vi "Open.vi"(7 "Allow multiple opens?":bool, 8 "error in (no error)":errorcluster, 10 "Channel Names":tag[](array[tag])) -> (0 "error out":errorcluster, 3 "AO (N Samples) Ref Out":T1)   [LabVIEW 2021, in "AO Block.lvlib"]
doc: "Opens a reference to analog output block write channel (ConnectorA/AO0). You must open a reference before you write values to the analog output block write channel."
uses:
  <vilib>/myRIO/Instrument Drivers/Onboard IO/AO Block/AO Block.lvlib
  <vilib>/myRIO/Instrument Drivers/Onboard IO/AO Block/typedefs/AO Block Reference.ctl
  <vilib>/myRIO/Common/Instrument Driver Framework/Utilities/typedefs/myRIO Generic Hardware Reference.ctl
  <vilib>/myRIO/Common/Instrument Driver Framework/Utilities/typedefs/Hardware Version Enum.ctl
  <vilib>/myRIO/Common/Instrument Driver Framework/Utilities/typedefs/myRIO v1.0 Reference.ctl
  <vilib>/myRIO/Common/Instrument Driver Framework/Utilities/typedefs/Generic FPGA Reference.ctl
  <vilib>/myRIO/Common/Instrument Driver Framework/myRIO v1.0/AO Block/typedefs/AO Block Channels List.ctl
  <vilib>/myRIO/Common/Instrument Driver Framework/myRIO v1.0/AO Block/typedefs/AO Block Channels Enum.ctl
  <vilib>/myRIO/Common/Instrument Driver Framework/Utilities/typedefs/Analog Scaling Constants.ctl
  <vilib>/userdefined/High Color/nirio_resource_hc.ctl
panel:
  # "AO (N Samples) Open"
  # "Opens a reference to the myRIO hardware and configures the AO Block Reference with channels to be written"
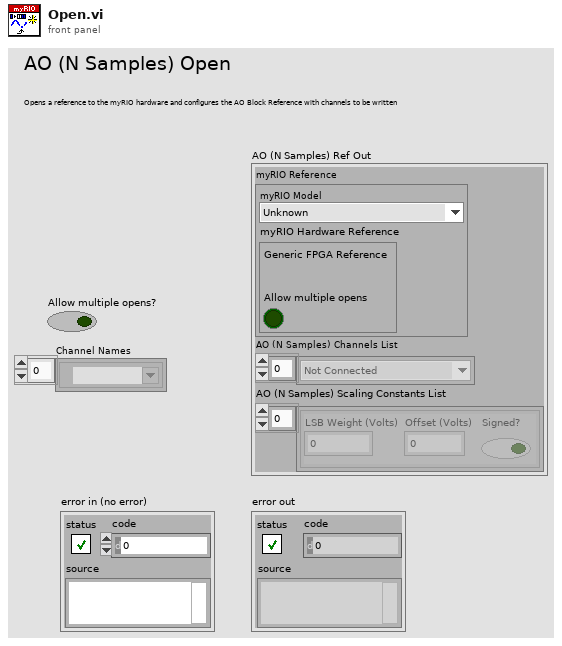
[diagram p1: front panel]
types:
  T1 = typedef "AO Block.lvlib/AO Block Reference.ctl" = cluster{"myRIO Reference":T2, "AO (N Samples) Channels List":T6, "AO (N Samples) Scaling Constants List":T8[]}
  T2 = typedef "myRIO Generic Hardware Reference.ctl" = cluster{"myRIO Model":T3, "myRIO Hardware Reference":T4}
  T3 = typedef "Hardware Version Enum.ctl" = enum16{"Unknown", "myRIO-1900", "myRIO-1950", "roboRIO", "NI ELVIS RIO CM", "ELVIS III"}
  T4 = typedef "myRIO v1.0 Reference.ctl" = cluster{"Generic FPGA Reference":T5, "Allow multiple opens":bool}
  T5 = typedef "Generic FPGA Reference.ctl" = refnum<k20>
  T6 = typedef "AO Block Channels List.ctl" = T7[]
  T7 = typedef "AO Block Channels Enum.ctl" = enum16{"Not Connected", "A/AO0 (N Samples)", "A/AO1 (N Samples)", "B/AO0 (N Samples)", "B/AO1 (N Samples)"}
  T8 = typedef "Analog Scaling Constants.ctl" = cluster{"LSB Weight (Volts)":dbl, "Offset (Volts)":dbl, "Signed?":bool}
  T9 = typedef "nirio_resource_hc.ctl" = tag
  T10 = typedef "Analog Scaling Constants List.ctl" = T8[]
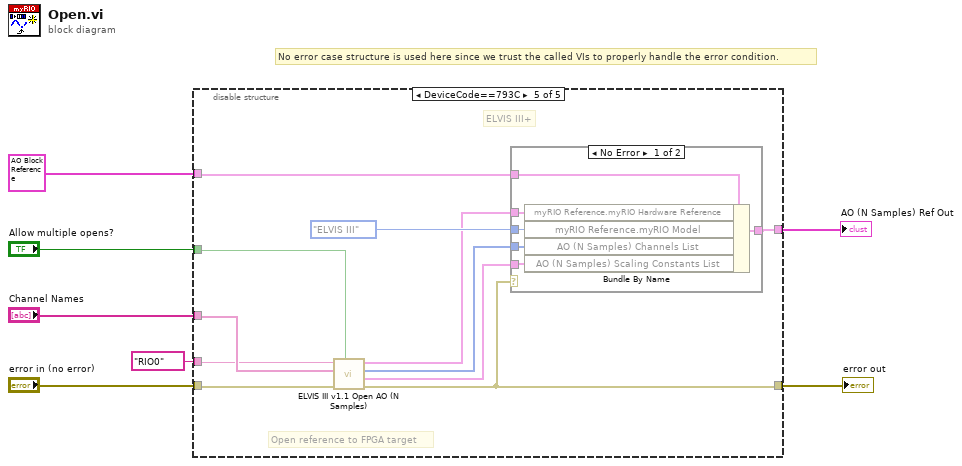
[diagram p0: block diagram]
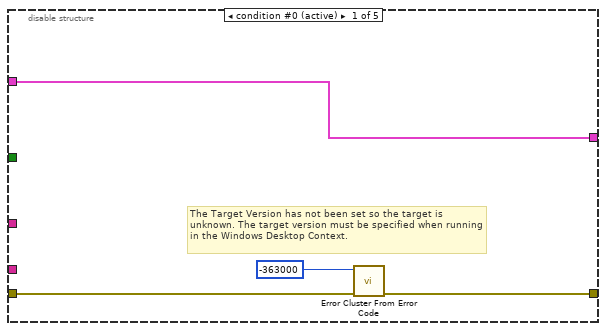
[diagram p2: hidden frame]
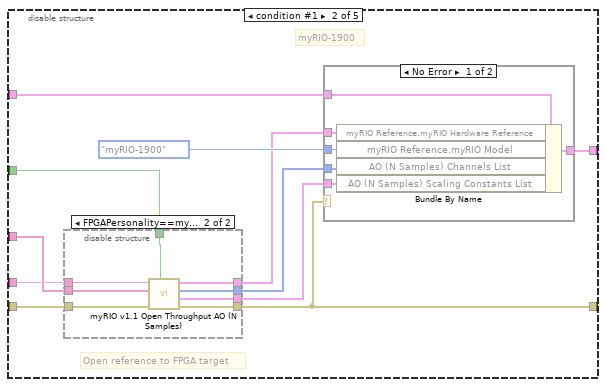
[diagram p3: hidden frame]
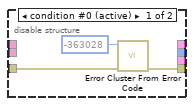
[diagram p4: hidden frame]
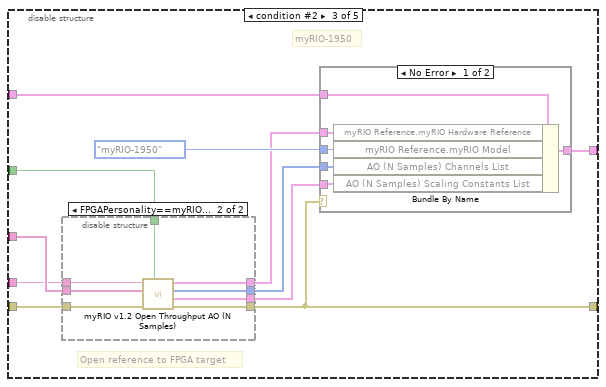
[diagram p6: hidden frame]
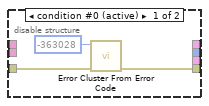
[diagram p7: hidden frame]
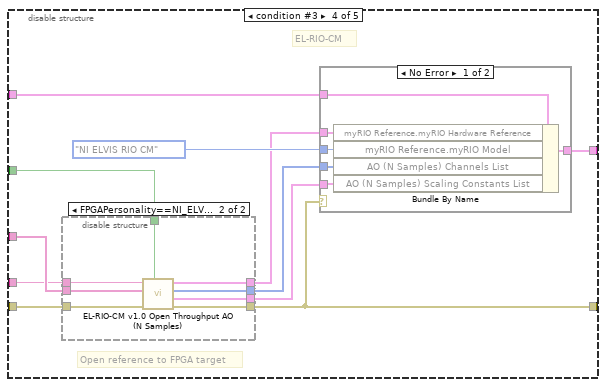
[diagram p9: hidden frame]
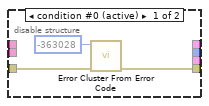
[diagram p10: hidden frame]
diagram:
  # "No error case structure is used here since we trust the called VIs to properly handle the error condition."
  n1 = disable-structure shown="DeviceCode==793C" {
    disable-tunnel: [w11 w14 w44 w73 w100] -> w5
    disable-tunnel: "Channel Names" -> [_ w22 w51 w80 w103]
    disable-tunnel: "Allow multiple opens?" -> [_ w18 w50 w79 w104]
    disable-tunnel: [w8 w21 w49 w78 w99] -> w4
    disable-tunnel: "error in (no error)" -> [w10 w19 w47 w76 w101]
    disable-tunnel: T1 {"myRIO Reference"={"myRIO Model"=enum."Unknown", "myRIO Hardware Reference"={"Generic FPGA Reference"=refnum, "Allow multiple opens"=FALSE}}, "AO (N Samples) Channels List"=[], "AO (N Samples) Scaling Constants List"=[]} ("AO (N Samples) Write Ref Out") -> [w8 w17 w46 w75 w105]
    disable-tunnel: T9 "RIO0" ("Resource name") -> [_ w15 w45 w74 w102]
    frame condition #0 (active) {
      # "The Target Version has not been set so the target is unknown. The target version must be specified when running in the Windows Desktop Context."
      n2 = call <vilib>:"Error Cluster From Error Code.vi"("error in (no error)"=w10, "error code (0)"=-363000) -> ("error out"=w11:errorcluster)  [unwired: 7 in]
    }
    frame condition #1 {
      # "myRIO-1900"
      # "Open reference to FPGA target"
      n3 = disable-structure shown="FPGAPersonality==myRIO_FP_Throughput" {
        disable-tunnel: w22 -> [_ w31]
        disable-tunnel: w19 -> [w24 w30]
        disable-tunnel: w18 -> [_ w33]
        disable-tunnel: [_ w28] -> w16
        disable-tunnel: w15 -> [_ w32]
        disable-tunnel: [w23 w26] -> w14
        disable-tunnel: [_ w29] -> w13
        disable-tunnel: [_ w27] -> w12
        frame condition #0 (active) {
          n4 = call <vilib>:"Error Cluster From Error Code.vi"("error in (no error)"=w24, "error code (0)"=-363028) -> ("error out"=w23:errorcluster)  [unwired: 7 in]
        }
        frame condition #1 {
          n5 = call <vilib>:"myRIO v1.1 Open Throughput AO (N Samples).vi"("Allow multiple opens?"=w33, "error in (no error)"=w30, "Channel Names"=w31, "Resource name"=w32) -> ("error out"=w26:errorcluster, "AO (N Samples) Scale Constants List"=w27:T10, "AO (N Samples) Channel List"=w28:T6, "myRIO Ref Out"=w29:T4)  [unwired: 4 in]
        }
      }
      n6 = case shown="No Error" w14 {
        tunnel: [w39 w40] -> w21
        tunnel: Hardware_Version_Enum."myRIO-1900" ("Hardware Version Enum") -> [w38 _]
        tunnel: w17 -> [w37 w40]
        tunnel: w16 -> [w36 _]
        tunnel: w13 -> [w35 _]
        tunnel: w12 -> [w34 _]
        frame No Error {
          n7 = Bundle By Name(cluster=w37, "myRIO Reference.myRIO Hardware Reference"=w35, "myRIO Reference.myRIO Model"=w38, "AO (N Samples) Channels List"=w36, "AO (N Samples) Scaling Constants List"=w34) -> (w39:T1)
        }
        frame Error {
        }
      }
    }
    frame condition #2 {
      # "myRIO-1950"
      # "Open reference to FPGA target"
      n8 = disable-structure shown="FPGAPersonality==myRIO_FP_Throughput" {
        disable-tunnel: w51 -> [_ w60]
        disable-tunnel: w50 -> [_ w62]
        disable-tunnel: w47 -> [w53 w59]
        disable-tunnel: w45 -> [_ w61]
        disable-tunnel: [w52 w55] -> w44
        disable-tunnel: [_ w58] -> w43
        disable-tunnel: [_ w57] -> w42
        disable-tunnel: [_ w56] -> w41
        frame condition #0 (active) {
          n9 = call <vilib>:"Error Cluster From Error Code.vi"("error in (no error)"=w53, "error code (0)"=-363028) -> ("error out"=w52:errorcluster)  [unwired: 7 in]
        }
        frame condition #1 {
          n10 = call <vilib>:"myRIO v1.2 Open Throughput AO (N Samples).vi"("Allow multiple opens?"=w62, "error in (no error)"=w59, "Channel Names"=w60, "Resource name"=w61) -> ("error out"=w55:errorcluster, "AO (N Samples) Scale Constants List"=w56:T10, "AO (N Samples) Channel List"=w57:T6, "myRIO Ref Out"=w58:T4)  [unwired: 4 in]
        }
      }
      n11 = case shown="No Error" w44 {
        tunnel: [w68 w69] -> w49
        tunnel: Hardware_Version_Enum."myRIO-1950" ("Hardware Version Enum") -> [w67 _]
        tunnel: w46 -> [w66 w69]
        tunnel: w43 -> [w65 _]
        tunnel: w42 -> [w64 _]
        tunnel: w41 -> [w63 _]
        frame No Error {
          n12 = Bundle By Name(cluster=w66, "myRIO Reference.myRIO Hardware Reference"=w65, "myRIO Reference.myRIO Model"=w67, "AO (N Samples) Channels List"=w64, "AO (N Samples) Scaling Constants List"=w63) -> (w68:T1)
        }
        frame Error {
        }
      }
    }
    frame condition #3 {
      # "EL-RIO-CM"
      # "Open reference to FPGA target"
      n13 = disable-structure shown="FPGAPersonality==NI_ELVIS_RIO_CM_FP_Throughput" {
        disable-tunnel: w80 -> [_ w89]
        disable-tunnel: w79 -> [_ w91]
        disable-tunnel: w76 -> [w82 w88]
        disable-tunnel: w74 -> [_ w90]
        disable-tunnel: [w81 w84] -> w73
        disable-tunnel: [_ w87] -> w72
        disable-tunnel: [_ w86] -> w71
        disable-tunnel: [_ w85] -> w70
        frame condition #0 (active) {
          n14 = call <vilib>:"Error Cluster From Error Code.vi"("error in (no error)"=w82, "error code (0)"=-363028) -> ("error out"=w81:errorcluster)  [unwired: 7 in]
        }
        frame condition #1 {
          n15 = call <vilib>:"EL-RIO-CM v1.0 Open Throughput AO (N Samples).vi"("Allow multiple opens?"=w91, "error in (no error)"=w88, "Channel Names"=w89, "Resource name"=w90) -> ("error out"=w84:errorcluster, "AO (N Samples) Scale Constants List"=w85:T10, "AO (N Samples) Channel List"=w86:T6, "myRIO Ref Out"=w87:T4)  [unwired: 4 in]
        }
      }
      n16 = case shown="No Error" w73 {
        tunnel: [w97 w98] -> w78
        tunnel: Hardware_Version_Enum."NI ELVIS RIO CM" ("Hardware Version Enum") -> [w96 _]
        tunnel: w75 -> [w95 w98]
        tunnel: w72 -> [w94 _]
        tunnel: w71 -> [w93 _]
        tunnel: w70 -> [w92 _]
        frame No Error {
          n17 = Bundle By Name(cluster=w95, "myRIO Reference.myRIO Hardware Reference"=w94, "myRIO Reference.myRIO Model"=w96, "AO (N Samples) Channels List"=w93, "AO (N Samples) Scaling Constants List"=w92) -> (w97:T1)
        }
        frame Error {
        }
      }
    }
    frame condition #4 {
      # "ELVIS III+"
      # "Open reference to FPGA target"
      n18 = call <vilib>:"ELVIS III v1.1 Open AO (N Samples).vi"("Allow multiple opens?"=w104, "error in (no error)"=w101, "Channel Names"=w103, "Resource name"=w102) -> ("error out"=w100:errorcluster, "AO (N Samples) Scale Constants List"=w106:T10, "AO (N Samples) Channel List"=w107:T6, "myRIO Ref Out"=w108:T4)  [unwired: 4 in]
      n19 = case shown="No Error" w100 {
        tunnel: [w115 w116] -> w99
        tunnel: Hardware_Version_Enum."ELVIS III" ("Hardware Version Enum") -> [w114 _]
        tunnel: w105 -> [w113 w116]
        tunnel: w108 -> [w112 _]
        tunnel: w107 -> [w111 _]
        tunnel: w106 -> [w110 _]
        frame No Error {
          n20 = Bundle By Name(cluster=w113, "myRIO Reference.myRIO Hardware Reference"=w112, "myRIO Reference.myRIO Model"=w114, "AO (N Samples) Channels List"=w111, "AO (N Samples) Scaling Constants List"=w110) -> (w115:T1)
        }
        frame Error {
        }
      }
    }
  }
  "AO (N Samples) Ref Out" <- w4
  "error out" <- w5
